vi "Counter-Single Pulse Output.vi"() -> ()   [LabVIEW 2011]
doc: "This example demonstrates how to generate a single pulse using a counter output. \n\nThe single pulse may be triggered once or repeatedly from an external source."
uses:
  <vilib>/Utility/error.llb/DialogType.ctl
  <vilib>/DAQmx/create/channels.llb/DAQmx Create Channel (CO-Pulse Generation-Time).vi
  <vilib>/DAQmx/configure/trigger.llb/DAQmx Start Trigger (Digital Edge).vi
  Program Files (x86)/National Instruments/LabVIEW 2011/resource/objmgr/daqmx.rc
panel:
  in  "milliseconds to wait":u32=100
  in  "stop":bool
  in  "Pulse Duration":dbl=0.001 format="%.6f"
  in  "Output Terminal":tag="/Dev1/PFI0"
  in  "Trigger Type":enum32{"No Trigger", "Digital Start"}(tab)
  in  "Retriggerable":bool
  in  "Edge":i32(ring)=10280 items=["Rising"=10280, "Falling"=10171]
  in  "Digital Trigger Source":tag
  in  "Stop":bool
  in  "Counter":tag="Dev1/ctr0"
  # "Channel Settings"
  # "Trigger Settings"
  # "To configure and use a trigger you must have the necessary tab selected above."
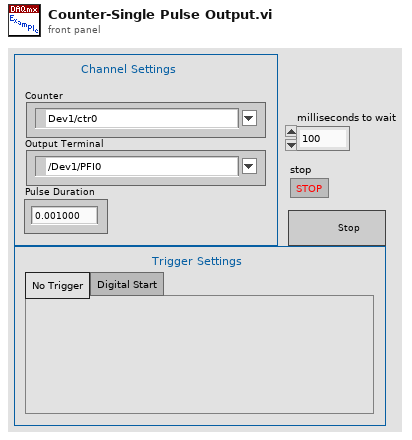
[diagram p1: front panel]
types:
  T1 = typedef "DialogType.ctl" = u16
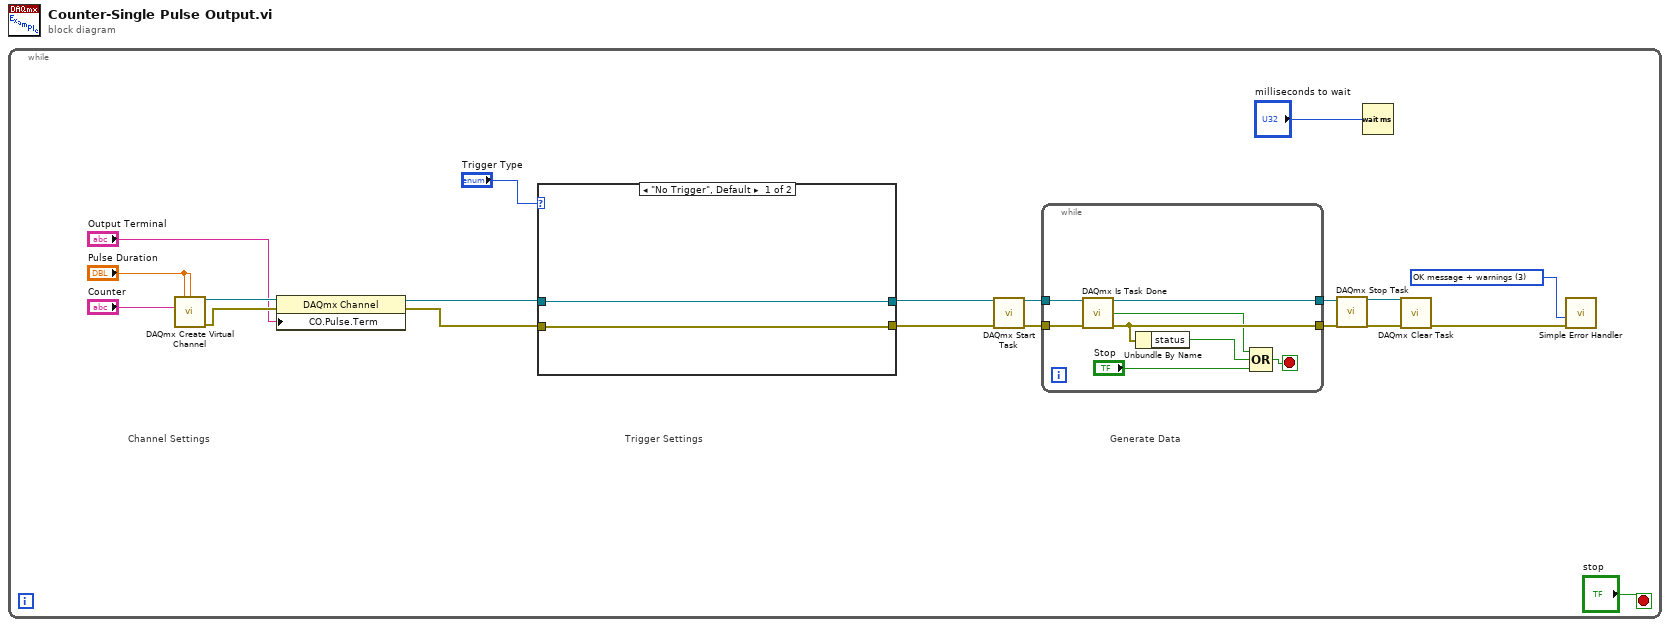
[diagram p0: block diagram]
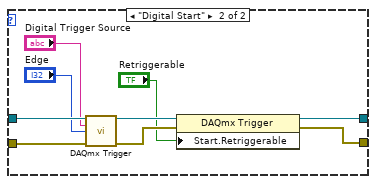
[diagram p2: hidden frame]
diagram:
  n1 = while {
    stop <- "stop" stop-if-true
    w3 = T1 3 items=["no dialog", "OK message", "continue or stop message", "OK message + warnings", "continue/stop + warnings"] ("type of dialog (OK msg:1)")
    # "Generate Data"
    # "Trigger Settings"
    # "Channel Settings"
    n2 = call-poly <vilib>:"DAQmx Create Virtual Channel.vi"("high time"="Pulse Duration", "low time"="Pulse Duration", "counter"="Counter") -> ("task out"=w13:refnum<k21>, "error out"=w12:errorcluster)  [unwired: 11 in]
    n3 = property class="DAQmx Channel"(reference=w13, error in=w12, "CO.Pulse.Term"="Output Terminal") -> (reference out=w9:refnum<k21>, error out=w10:errorcluster)
    n4 = case shown="\"No Trigger\", Default" "Trigger Type" {
      tunnel: w9 -> [w30 w39]
      tunnel: w10 -> [w29 w38]
      tunnel: [w30 w35] -> w14
      tunnel: [w29 w34] -> w15
      frame "No Trigger", Default {
      }
      frame "Digital Start" {
        n5 = call-poly <vilib>:"DAQmx Trigger.vi"("task/channels in"=w39, "source"="Digital Trigger Source", "edge"="Edge", "error in"=w38) -> ("task out"=w32:refnum<k21>, "error out"=w33:errorcluster)  [unwired: 10 in]
        n6 = property class="DAQmx Trigger"(reference=w32, error in=w33, "Start.Retriggerable"="Retriggerable") -> (reference out=w35:refnum<k21>, error out=w34:errorcluster)
      }
    }
    n7 = call <vilib>:"DAQmx Start Task.vi"("task/channels in"=w14, "error in"=w15) -> ("task out"=w20:refnum<k21>, "error out"=w19:errorcluster)  [unwired: 12 in]
    n8 = while {
      tunnel: w20 -> [w28]
      tunnel: w19 -> [w27]
      tunnel: [w24] -> w6
      tunnel: [w25] -> w7
      stop <- w26 stop-if-true
      n9 = call <vilib>:"DAQmx Is Task Done.vi"("task/channels in"=w28, "error in"=w27) -> ("task out"=w25:refnum<k21>, "task done?"=w21:bool, "error out"=w24:errorcluster)  [unwired: 11 in]
      n10 = Unbundle By Name(w24) -> ("status"=w23:bool)
      n11 = Compound Arithmetic op=OR(w21, w23, "Stop") -> (w26:bool)
    }
    n12 = call <vilib>:"DAQmx Stop Task.vi"("task/channels in"=w7, "error in"=w6) -> ("task out"=w5:refnum<k21>, "error out"=w4:errorcluster)  [unwired: 12 in]
    n13 = Wait (ms)(milliseconds to wait="milliseconds to wait") -> ()  [unwired: 1 out]
    n14 = call <vilib>:"DAQmx Clear Task.vi"("task in"=w5, "error in"=w4) -> ("error out"=w18:errorcluster)  [unwired: 13 in]
    n15 = call <vilib>:"Simple Error Handler.vi"("type of dialog (OK msg:1)"=w3, "error in (no error)"=w18) -> ()  [unwired: 3 in, 5 out]
  }
